vi "RT - Read Config.vi"(8 "error in":errorcluster, 10 "CONFIG STRING":T1={"BODY CAL"=["TWTT OP (IN)", "TWTT PDP (IN)", "DLT OP (IN)", "DLT PDP 01 (IN)", "DLT PDP 02 (IN)", "BR OP (IN)", "BR TWT ALIGN", "BR DL ALIGN (IN)"], "US CAL"=["HPL Low (PSI)", "HPL High (PSI)", "HPH Low (PSI)", "HPH High (PSI)", "AP Low (PSI)", "AP High (PSI)", "DL Clean (SEC)", "Reset (MIN)"]}, 11 "ConfigFile Path In":path) -> (0 "error out":errorcluster, 2 "US CAL":dbl[](array[numeric]), 3 "BODY CAL":dbl[](array[numeric]))   [LabVIEW 2018]
uses:
  Controls/ConfigString.ctl
  <vilib>/Utility/config.llb/Read Key (Double).vi
  <vilib>/Utility/config.llb/NI_LVConfig.lvlib
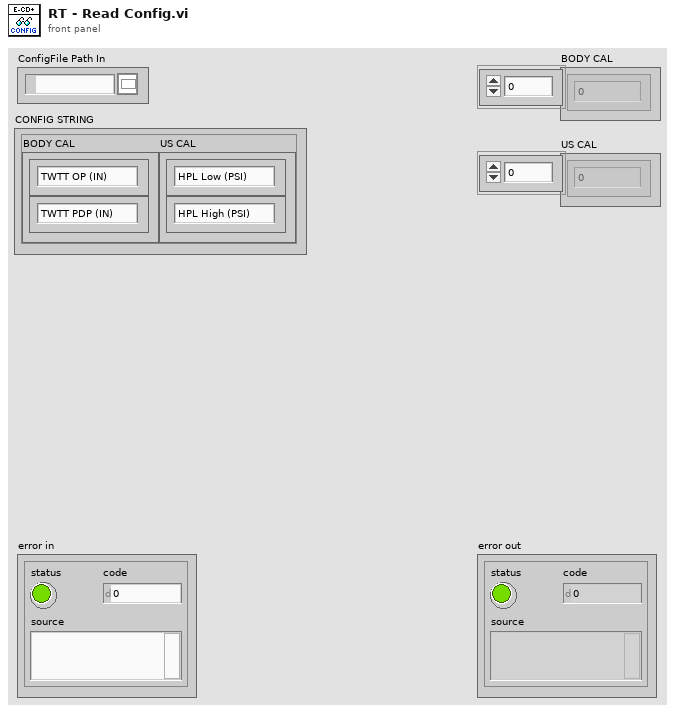
[diagram p1: front panel]
types:
  T1 = typedef "ConfigString.ctl" = cluster{"BODY CAL":string[], "US CAL":string[]}
  T2 = typedef "NI_LVConfig.lvlib/Config Data RefNum.ctl" = refnum<k1>
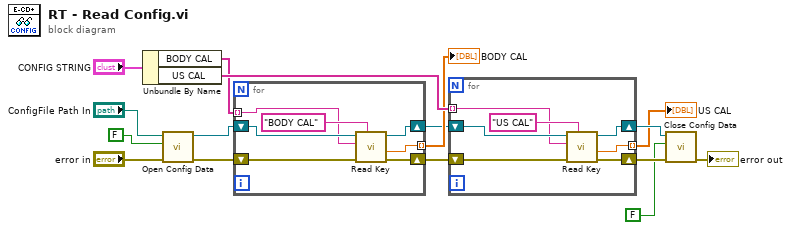
[diagram p0: block diagram]
diagram:
  n1 = Unbundle By Name("CONFIG STRING") -> ("BODY CAL"=w14:string[], "US CAL"=w15:string[])
  n2 = call <vilib>:"Open Config Data.vi"("error in (no error)"="error in", "create file if necessary (T)"=FALSE, "configuration file path"="ConfigFile Path In") -> ("error out"=w5:errorcluster, "refnum"=w6:T2)  [unwired: 6 in, 1 out]
  n3 = for {
    tunnel: w14 -> [w20] mode=indexing
    shift-right: [w19] -> w8
    shift-left: w6 -> [w22]
    shift-right: [w18] -> w9
    shift-left: w5 -> [w23]
    tunnel: [w17] -> w10 mode=indexing
    n4 = call-poly <vilib>:"Read Key.vi"("section"="BODY CAL", "error in (no error)"=w23, "key"=w20, "refnum"=w22) -> ("error out"=w18:errorcluster, "value"=w17:dbl, "refnum out"=w19:T2)  [unwired: 4 in, 1 out]
  }
  "BODY CAL" <- w10
  n5 = for {
    tunnel: w15 -> [w27] mode=indexing
    shift-right: [w26] -> w12
    shift-left: w8 -> [w29]
    shift-right: [w25] -> w13
    shift-left: w9 -> [w30]
    tunnel: [w24] -> w11 mode=indexing
    n6 = call-poly <vilib>:"Read Key.vi"("section"="US CAL", "error in (no error)"=w30, "key"=w27, "refnum"=w29) -> ("error out"=w25:errorcluster, "value"=w24:dbl, "refnum out"=w26:T2)  [unwired: 4 in, 1 out]
  }
  "US CAL" <- w11
  n7 = call <vilib>:"Close Config Data.vi"("error in (no error)"=w13, "write file if changed (T)"=FALSE, "refnum"=w12) -> ("error out"=→"error out":errorcluster)  [unwired: 8 out]
